vi "Calculate Forces.vi"(7 "Integrator Reset":bool, 8 "error in (no error)":errorcluster, 10 "Vessel in":refnum<class "Vessel.lvclass">, 11 "Controller in":refnum<class "Controller.lvclass">) -> (0 "error out":errorcluster, 2 "Vessel out":refnum<class "Vessel.lvclass">, 3 "Controller out":refnum<class "Controller.lvclass">)   [LabVIEW 2014, in "Controller Library.lvlib" / "Controller.lvclass"]
doc: "This VI calculates the forces in each controlled degree of freedom direction to follow a desired path or point."
uses:
  Controller.lvclass
  ROV/Vessel.lvclass
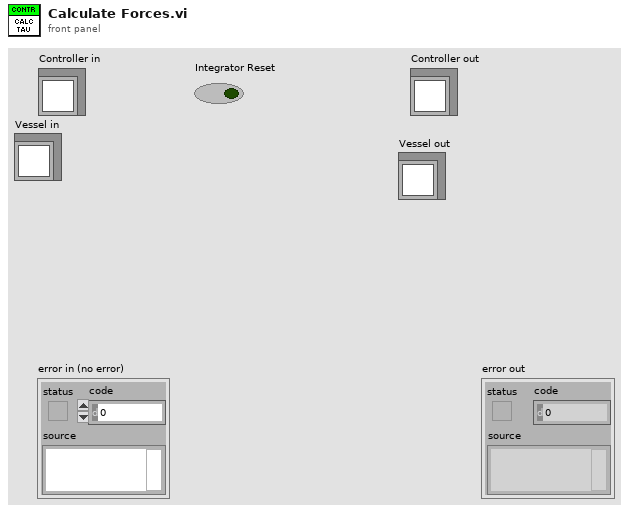
[diagram p1: front panel]
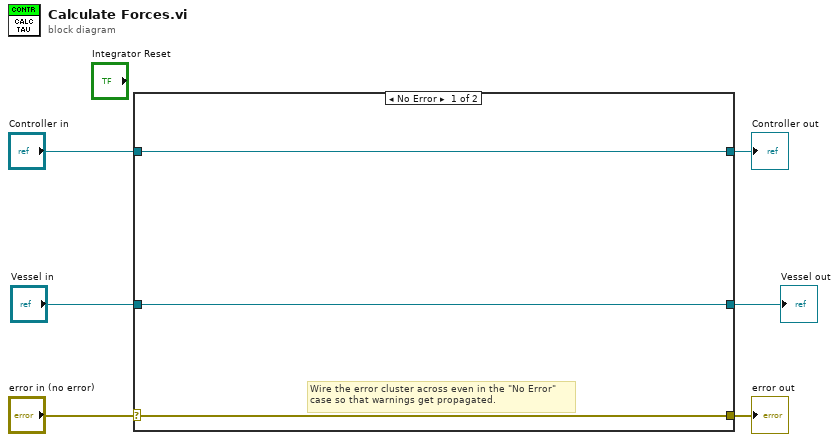
[diagram p0: block diagram]
diagram:
  n1 = case shown="No Error" "error in (no error)" {
    selector: "error in (no error)" -> [w8 w12]
    tunnel: [w8 w12] -> w5
    tunnel: [w9 w11] -> w3
    tunnel: "Controller in" -> [w9 w11]
    tunnel: "Vessel in" -> [w7 w10]
    tunnel: [w7 w10] -> w1
    frame No Error {
      # "Wire the error cluster across even in the \"No Error\"\ncase so that warnings get propagated."
    }
    frame Error {
    }
  }
  "error out" <- w5
  "Controller out" <- w3
  "Vessel out" <- w1
